vi "Write Log Scan Progress.vi"(8 "error in (no error)":errorcluster, 10 "Scan Progress":T1 {"Actuator Data"."Timestamp" format="%.4f"; "Actuator Data"."Force" format="%.4f"}, 11 "Model in":refnum<class "Model.lvclass">) -> (0 "error out":errorcluster, 3 "Model out":refnum<class "Model.lvclass">)   [LabVIEW 2016]
uses:
  Test Log/Test Log/Test Log.lvclass
  Model.lvclass
  Typedefs/ScanProgress.ctl
  Typedefs/HPMT_Typedefs.lvlib
  Typedefs/ActuatorData.ctl
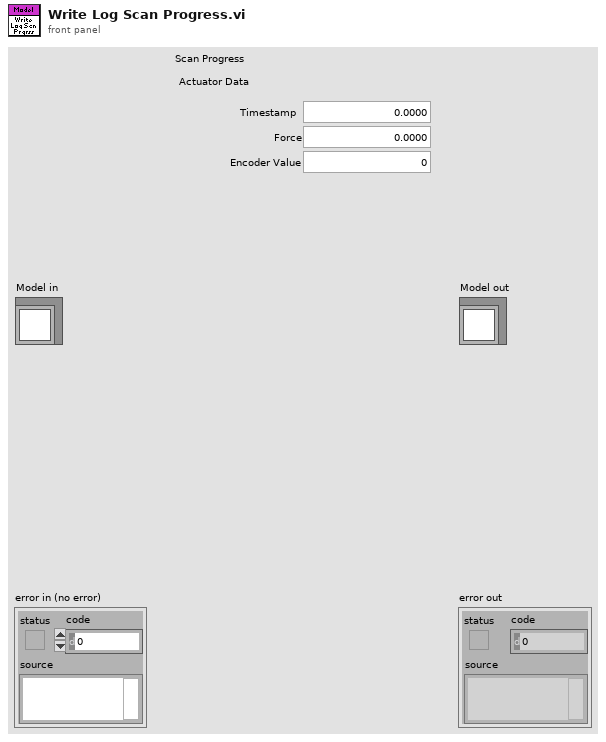
[diagram p1: front panel]
types:
  T1 = typedef "HPMT_Typedefs.lvlib/ScanProgress.ctl" = cluster{"Actuator Data":T2}
  T2 = typedef "HPMT_Typedefs.lvlib/ActuatorData.ctl" = cluster{"Timestamp":dbl, "Force":dbl, "Encoder Value":i32}
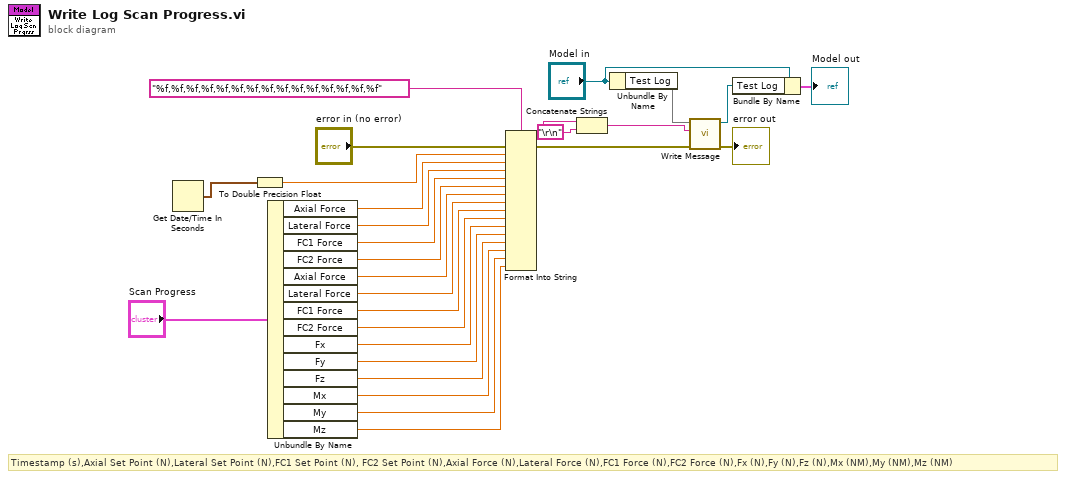
[diagram p0: block diagram]
diagram:
  # "Timestamp (s),Axial Set Point (N),Lateral Set Point (N),FC1 Set Point (N), FC2 Set Point (N),Axial Force (N),Lateral Force (N),FC1 Force (N),FC2 Force (N),Fx (N),Fy (N),Fz (N),Mx (NM),My (NM),Mz (NM)"
  n1 = Get Date/Time In Seconds() -> (seconds since 1Jan1904=w21:timestamp)
  n2 = To Double Precision Float(number=w21) -> (double precision float=w20:dbl)
  n3 = Unbundle By Name("Scan Progress") -> ("Axial Force"=w14:dbl, "Lateral Force"=w13:dbl, "FC1 Force"=w12:dbl, "FC2 Force"=w11:dbl, "Axial Force"=w10:dbl, "Lateral Force"=w9:dbl, "FC1 Force"=w8:dbl, "FC2 Force"=w7:dbl, "Fx"=w6:dbl, "Fy"=w5:dbl, "Fz"=w4:dbl, "Mx"=w3:dbl, "My"=w2:dbl, "Mz"=w1:dbl)
  n4 = Format Into String(format string="%f,%f,%f,%f,%f,%f,%f,%f,%f,%f,%f,%f,%f,%f,%f", error in="error in (no error)", w20, w14, w13, w12, w11, w10, w9, w8, w7, w6, w5, w4, w3, w2, w1) -> (resulting string=w17:string, error out=w24:errorcluster)  [unwired: 1 in]
  n5 = Concatenate Strings(w17, "\r\n") -> (w16:string)
  n6 = Unbundle By Name("Model in") -> ("Test Log"=w22)
  n7 = call-dynamic "Write Message.vi"("error in (no error)"=w24, "Message"=w16, "Test Log in"=w22) -> ("error out"=→"error out":errorcluster, "Test Log out"=w25:refnum<class "Test Log.lvclass">)  [unwired: 7 in]
  n8 = Bundle By Name(cluster="Model in", "Test Log"=w25) -> (→"Model out":cluster{})
